vi "gentec-M-Link.Get Waveform Averages.vi"(0 "VISA resource In":refnum<visa-resource-name>, 5 "error in (no error)":errorcluster) -> (11 "Data Read":string, 13 "Read Timeout":bool, 14 "VISA resource Out":refnum<visa-resource-name>, 16 "Waveform Averages":T1 items=["None", "2", "4", "8", "16", "32", "64", "128"], 19 "error out":errorcluster)   [LabVIEW 2014, in "gentec-M-Link - Driver.lvlib"]
doc: "Data to write: avg\n\nQueries the sampling size of the noise suppression."
uses:
  gentec-M-Link - Driver.lvlib
  Type Defs/gentec-M-Link.Waveform Averages.ctl
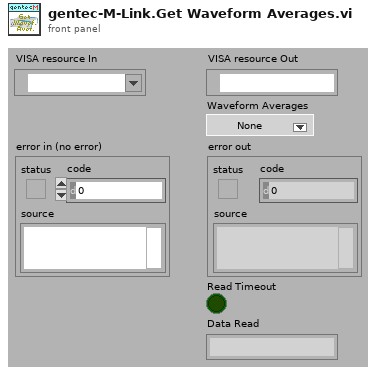
[diagram p1: front panel]
types:
  T1 = typedef "gentec-M-Link - Driver.lvlib/gentec-M-Link.Waveform Averages.ctl" = u16
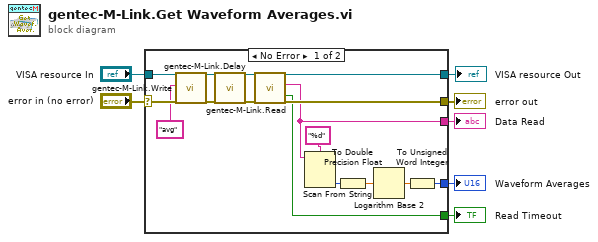
[diagram p0: block diagram]
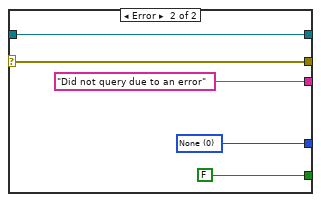
[diagram p2: hidden frame]
diagram:
  n1 = case shown="No Error" "error in (no error)" {
    selector: "error in (no error)" -> [w20 w28]
    tunnel: [w21 w28] -> w6
    tunnel: "VISA resource In" -> [w19 w27]
    tunnel: [w18 w27] -> w4
    tunnel: [w9 w24] -> w3
    tunnel: [w13 "Did not query due to an error" ("Data Read")] -> w2
    tunnel: [w14 FALSE ("Read Timeout")] -> w1
    frame No Error {
      n2 = call "gentec-M-Link.Write.vi"("VISA resource (In)"=w19, "Data To Write"="avg", "error in (no error)"=w20) -> ("VISA resource (Out)"=w23:refnum<visa-resource-name>, "error out"=w22:errorcluster)  [unwired: 14 in, 1 out]
      n3 = call "gentec-M-Link.Delay.vi"("VISA resource In"=w23, "error in (no error)"=w22) -> ("VISA resource Out"=w17:refnum<visa-resource-name>, "error out"=w16:errorcluster)  [unwired: 16 in]
      n4 = call "gentec-M-Link.Read.vi"("VISA resource (In)"=w17, "error in (no error)"=w16) -> ("VISA resource (Out)"=w18:refnum<visa-resource-name>, "Data Read"=w13:string, "Read Timeout"=w14:bool, "error out"=w21:errorcluster)  [unwired: 13 in, 1 out]
      n5 = Scan From String(format string="%d", input string=w13) -> (output 1=w11:i32)  [unwired: 3 in, 3 out]
      n6 = To Double Precision Float(number=w11) -> (double precision float=w8:dbl)
      n7 = Logarithm Base 2(1:w8) -> (0:w10:dbl)
      n8 = To Unsigned Word Integer(number=w10) -> (unsigned 16bit integer=w9:u16)
    }
    frame Error {
      w24 = T1 0 items=["None", "2", "4", "8", "16", "32", "64", "128"] ("Waveform Averages")
    }
  }
  "error out" <- w6
  "VISA resource Out" <- w4
  "Waveform Averages" <- w3
  "Data Read" <- w2
  "Read Timeout" <- w1
